vi "Initialize.vi"(8 "error in (no error)":errorcluster, 9 "Calling VI":refnum<vi>, 10 "UI Display":refnum<vi>, 11 "LabVIEW Build Script in":refnum<class "LabVIEW Build Script.lvclass">) -> (0 "error out":errorcluster, 3 "LabVIEW Build Script out":refnum<class "LabVIEW Build Script.lvclass">)   [LabVIEW 2021, in "LabVIEW Build Script.lvclass"]
uses:
  LabVIEW Build Script.lvclass
  LabVIEW Build Script.lvclass/LabVIEW Build Script.ctl
  Build Script Common/Build Script Common.lvlib
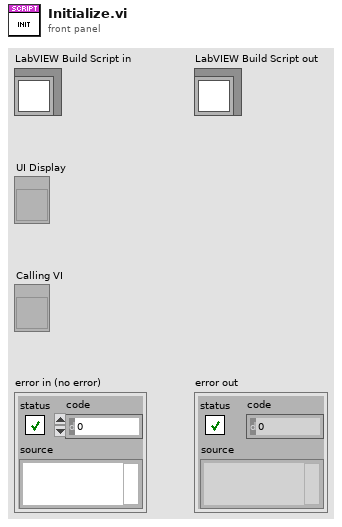
[diagram p1: front panel]
types:
  T1 = typedef "Build Script Common.lvlib/References.ctl" = cluster{"UI Display":refnum<vi>, "UI Display Valid":bool, "UI Semaphore":T2}
  T2 = typedef "Semaphore RefNum" = refnum<k1>
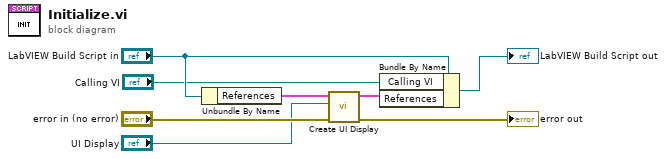
[diagram p0: block diagram]
diagram:
  n1 = Unbundle By Name("LabVIEW Build Script in") -> ("References"=w6:T1)
  n2 = call "Create UI Display.vi"("error in (no error)"="error in (no error)", "UI Display"="UI Display", "References in"=w6) -> ("error out"=→"error out":errorcluster, "References out"=w4:T1)  [unwired: 7 in]
  n3 = Bundle By Name(cluster="LabVIEW Build Script in", "Calling VI"="Calling VI", "References"=w4) -> (→"LabVIEW Build Script out":refnum<class "LabVIEW Build Script.lvclass">)
